vi "update.vi"(8 "error in (no error)":errorcluster, 11 "TrajectoryMG100122AODFrameScan in":refnum<class "TrajectoryMH100122AODRAPS.lvclass">) -> (0 "error out":errorcluster, 3 "TrajectoryMG100122AODFrameScan out":refnum<class "TrajectoryMH100122AODRAPS.lvclass">)   [LabVIEW 2010, in "TrajectoryMH100122AODRAPS.lvclass"]
uses:
  TrajectoryMH100122AODRAPS.lvclass
  FPGAWrapper/FPGAWrapperMH120124AOD/FPGAWrapperMH120124RAPS_PXI7813R/FPGAWrapperMH120124RAPS_PXI7813R.lvclass
  FPGAWrapper/GenericFPGAWrapper/GenericFPGAWrapper/GenericFPGAWrapper.lvclass
  common/classes/GenericComponent/GenericComponent/class_data.vi
  common/classes/GenericComponent/GenericComponent/GenericComponent.lvclass
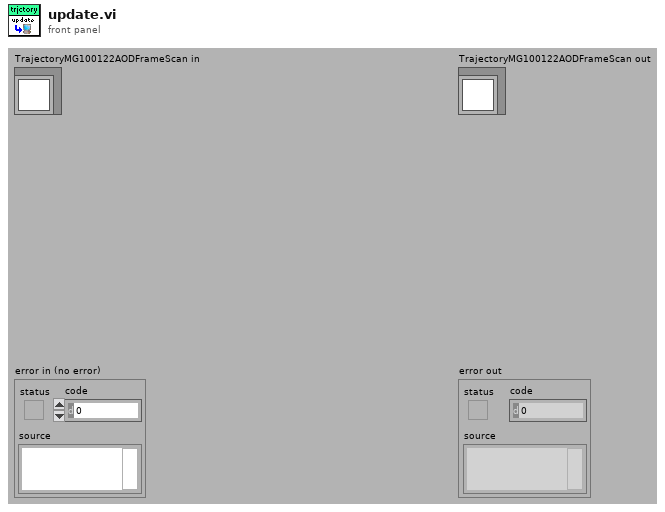
[diagram p1: front panel]
types:
  T1 = typedef "FPGAWrapperMH120124RAPS_PXI7813R.lvclass/raps_point_cluster.ctl" = cluster{"x":u16, "y":u16, "z":u16, "amplitude":u16}
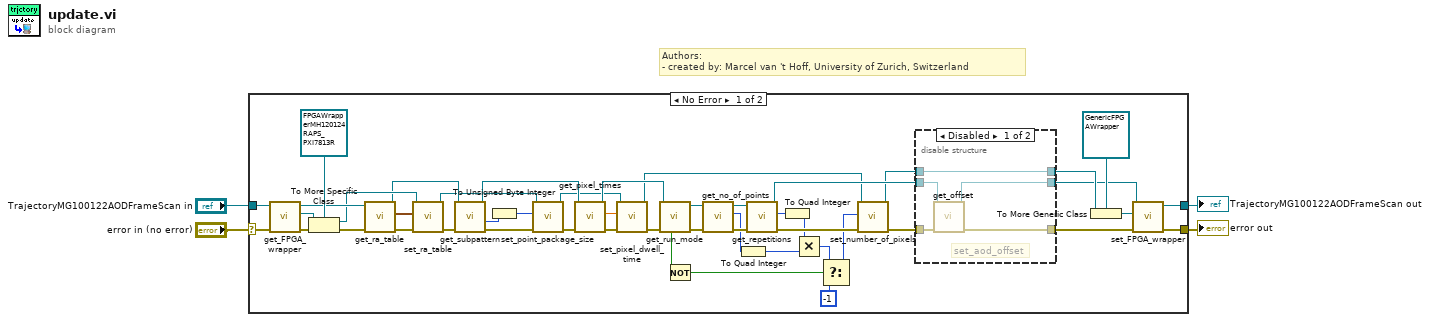
[diagram p0: block diagram]
diagram:
  # "Authors: \n- created by: Marcel van 't Hoff, University of Zurich, Switzerland"
  n1 = case shown="No Error" "error in (no error)" {
    selector: "error in (no error)" -> [w46 w62]
    tunnel: [w51 w62] -> w4
    tunnel: "TrajectoryMG100122AODFrameScan in" -> [w45 w61]
    tunnel: [w50 w61] -> w3
    frame No Error {
      n2 = call-dynamic "get_FPGA_wrapper.vi"("error in (no error)"=w46, "TrajectoryMG100122GenericFPGA in"=w45) -> ("error out"=w44:errorcluster, "GenericFPGAWrapper.lvclass"=w47:refnum<class "GenericFPGAWrapper.lvclass">, "TrajectoryMG100122GenericFPGA out"=w22:refnum<class "TrajectoryMH100122AODRAPS.lvclass">)  [unwired: 7 in]
      n3 = To More Specific Class(target class=refnum<class "FPGAWrapperMH120124RAPS_PXI7813R.lvclass"> refnum ("FPGAWrapperMH120124RAPS_PXI7813R.lvclass"), reference=w47, error in=w44) -> (specific class reference=w21:refnum<class "FPGAWrapperMH120124RAPS_PXI7813R.lvclass">, error out=w20:errorcluster)
      n4 = call-dynamic "get_ra_table.vi"("error in (no error)"=w20, "TrajectoryMH100122AODRAPS in"=w22) -> ("error out"=w43:errorcluster, "RAPS points"=w19:T1[], "TrajectoryMH100122AODRAPS out"=w10:refnum<class "TrajectoryMH100122AODRAPS.lvclass">)  [unwired: 7 in]
      n5 = call-dynamic "set_ra_table.vi"("error in (no error)"=w43, "RAPS points"=w19, "FPGAWrapperMH120124RAPS_PXI7813R in"=w21) -> ("error out"=w12:errorcluster, "FPGAWrapperMH120124RAPS_PXI7813R out"=w8:refnum<class "FPGAWrapperMH120124RAPS_PXI7813R.lvclass">)  [unwired: 7 in]
      n6 = call-dynamic "get_subpattern.vi"("error in (no error)"=w12, "TrajectoryMH100122AODRAPS in"=w10) -> ("error out"=w11:errorcluster, "number of iteration points"=w6:i32, "TrajectoryMH100122AODRAPS out"=w9:refnum<class "TrajectoryMH100122AODRAPS.lvclass">)  [unwired: 4 in, 3 out]
      n7 = To Unsigned Byte Integer(number=w6) -> (unsigned 8bit integer=w5:u8)
      n8 = call "set_point_package_size.vi"("error in (no error)"=w11, "point package size"=w5, "FPGAWrapperMH120124RAPS_PXI7813R in"=w8) -> ("error out"=w13:errorcluster, "FPGAWrapperMH120124RAPS_PXI7813R out"=w7:refnum<class "FPGAWrapperMH120124RAPS_PXI7813R.lvclass">)  [unwired: 7 in]
      n9 = call-dynamic "get_pixel_times.vi"("error in (no error)"=w13, "TrajectoryMG100122AODFrameScan in"=w9) -> ("error out"=w52:errorcluster, "acquisition time"=w38:dbl[unit], "TrajectoryMG100122AODFrameScan out"=w23:refnum<class "TrajectoryMH100122AODRAPS.lvclass">)  [unwired: 5 in, 2 out]
      n10 = call-dynamic "set_pixel_dwell_time.vi"("error in (no error)"=w52, "pixel dwell time"=w38, "FPGAWrapperMH120124RAPS_PXI7813R in"=w7) -> ("error out"=w18:errorcluster, "FPGAWrapperMH120124RAPS_PXI7813R out"=w17:refnum<class "FPGAWrapperMH120124RAPS_PXI7813R.lvclass">)  [unwired: 7 in]
      n11 = call "get_run_mode.vi"("error in (no error)"=w18, "GenericPlugin in"=w23) -> ("error out"=w30:errorcluster, "GenericPlugin out"=w31:refnum<class "TrajectoryMH100122AODRAPS.lvclass">, "is free run?"=w27:bool)  [unwired: 5 in, 2 out]
      n12 = Not(x=w27) -> (.not. x?=w26:bool)
      n13 = call-dynamic "get_no_of_points.vi"("error in (no error)"=w30, "TrajectoryMH100122AODRAPS in"=w31) -> ("error out"=w37:errorcluster, "no. of points"=w35:i32, "TrajectoryMH100122AODRAPS out"=w34:refnum<class "TrajectoryMH100122AODRAPS.lvclass">)  [unwired: 7 in]
      n14 = To Quad Integer(1:w35) -> (0:w16:i64)
      n15 = call-dynamic "get_repetitions.vi"("error in (no error)"=w37, "GenericTrajectory in"=w34) -> ("error out"=w36:errorcluster, "repetitions"=w32:i32, "GenericTrajectory out"=w33:refnum<class "TrajectoryMH100122AODRAPS.lvclass">)  [unwired: 7 in]
      n16 = To Quad Integer(1:w32) -> (0:w25:i64)
      n17 = Multiply(x=w25, y=w16) -> (x*y=w24:i64)
      n18 = Select(t=w24, s=w26, f=i64 -1 ("t")) -> (s? t:f=w29:i64)
      n19 = call-dynamic "set_number_of_pixels.vi"("error in (no error)"=w36, "number of pixels"=w29, "FPGAWrapperMH120124RAPS_PXI7813R in"=w17) -> ("error out"=w14:errorcluster, "FPGAWrapperMH120124RAPS_PXI7813R out"=w15:refnum<class "FPGAWrapperMH120124RAPS_PXI7813R.lvclass">)  [unwired: 7 in]
      n20 = disable-structure shown="Disabled" {
        disable-tunnel: w15 -> [w55 w58]
        disable-tunnel: w33 -> [w57 w59]
        disable-tunnel: w14 -> [w56 w60]
        disable-tunnel: [w53 w60] -> w39
        disable-tunnel: [w54 w59] -> w40
        disable-tunnel: [w55 w58] -> w41
        frame Disabled {
          # "set_aod_offset"
          n21 = call-dynamic "get_offset.vi"("error in (no error)"=w56, "TrajectoryMH100122AODRAPS in"=w57) -> ("error out"=w53:errorcluster, "TrajectoryMH100122AODRAPS out"=w54:refnum<class "TrajectoryMH100122AODRAPS.lvclass">)  [unwired: 7 in, 1 out]
        }
        frame Enabled {
        }
      }
      n22 = To More Generic Class(target class=refnum<class "GenericFPGAWrapper.lvclass"> refnum ("GenericFPGAWrapper.lvclass"), reference=w41) -> (generic class reference=w48:refnum<class "GenericFPGAWrapper.lvclass">)
      n23 = call-dynamic "set_FPGA_wrapper.vi"("error in (no error)"=w39, "GenericFPGAWrapper.lvclass"=w48, "TrajectoryMG100122GenericFPGA in"=w40) -> ("error out"=w51:errorcluster, "TrajectoryMG100122GenericFPGA out"=w50:refnum<class "TrajectoryMH100122AODRAPS.lvclass">)  [unwired: 7 in]
    }
    frame Error {
    }
  }
  "error out" <- w4
  "TrajectoryMG100122AODFrameScan out" <- w3
